vi "modulation signal.vi"() -> ()   [LabVIEW 2021]
panel:
  out "Waveform Graph":dynamicdata(graph)
  out "message":dynamicdata(graph)
  out "modulator":dynamicdata(graph)
  out "carrier":dynamicdata(graph)
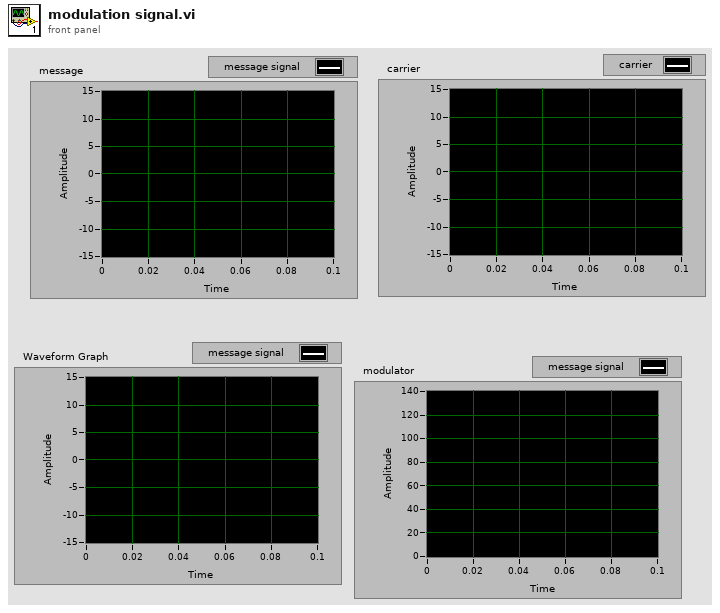
[diagram p1: front panel]
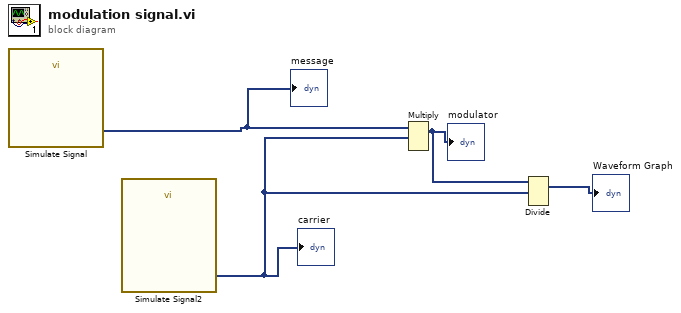
[diagram p0: block diagram]
diagram:
  n1 = call "Simulate Signal"() -> ("message signal"=w4:dynamicdata)  [unwired: 14 in, 1 out]
  "message" <- w4
  n2 = call "Simulate Signal2"() -> ("carrier"=w2:dynamicdata)  [unwired: 14 in, 1 out]
  "carrier" <- w2
  n3 = Multiply(1:w2, 2:w4) -> (0:w3:dynamicdata)  [unwired: 1 in, 1 out]
  "modulator" <- w3
  n4 = Divide(1:w2, 2:w3) -> (0:→"Waveform Graph":dynamicdata)  [unwired: 1 in, 1 out]
